vi "AprilTag Target Package Rebound Rumble Code.vi"() -> ()   [LabVIEW 2023]
uses:
  <vilib>/vision/Image Controls.llb/IMAQ Image.ctl
  <vilib>/Utility/config.llb/NI_LVConfig.lvlib
  Camera Set Up/Event/Event Setup Types.ctl
  State Machine/AprialTag States.ctl
  State Machine/AprialTag Main Cluster.ctl
  Steam Type.ctl
  <vilib>/Utility/config.llb/Write Key (String).vi
  <vilib>/Utility/config.llb/Read Key (String).vi
  <vilib>/ptbypt/NI_PtbyPt.lvlib
  <vilib>/vision/NI_Vision_Development_Module.lvlib
  Camera Info.ctl
  <vilib>/vision/Pattern Matching.llb/IMAQ Match Range Setting.ctl
  <vilib>/vision/Shape Detection.llb/ShapeDetectionMatchOptions.ctl
panel:
  in  "Main":enum32{"Page 1", "Page 2"}(tab)
  out "Target Pitch":dbl[](array[numeric]) caption="Tag Pitch (deg)" format="%.1f"
  out "Target Yaw":dbl[](array[numeric]) caption="Tag Yaw (deg)" format="%.1f"
  out "Tag ID":dbl[](array[numeric]) caption="Tag Number"
  out "Image":T1(plugin-control)
  in  "Camera Name":string="cam0"
  in  "Settings":bool
  in  "Save":bool
  in  "Tools":bool
  out "AprilTag Fps":dbl format="%#.0f"
  out "Distance":dbl[](array[numeric]) caption="Tag Distance (in)" format="%.1f"
  out "Angle":dbl[](array[numeric]) caption="Center Angle (deg)" format="%.1f"
  in  "Minimum match score":dbl=100.0
  in  "Home":bool
  in  "Robot Calibration Cluster":T2={"Camera Height on robot (in)"=9.5, "Camera Angle on the robot (deg)"=2.5, "Camera FOV Top to Bottom View Angle (deg)"=26.5, "Camera FOV Left to Right View Angle (deg)"=68.5, "Target size (in)"=6.5, "Distance to front of bumper (in)"=9.75, "Focal Length (mm)"=10.0, "Yaw Slope"=12.276, "Yaw Offset"=2.0} {"Yaw Offset" format="%#_13g"; "Yaw Slope" format="%#_13g"; "Camera FOV Left to Right View Angle (deg)" format="%#_13g"; "Focal Length (mm)" format="%#_13g"; "Distance to front of bumper (in)" format="%#_13g"; "Target size (in)" format="%#_13g"; "Camera FOV Top to Bottom View Angle (deg)" format="%#_13g"; "Camera Angle on the robot (deg)" format="%#_13g"; "Camera Height on robot (in)" format="%#_13g"}
  in  "Max Rect Size (pix)":dbl=1200.0
  in  "Min Rect Size (pix)":dbl=50.0
  in  "Match Options":T3={"Rotation"=TRUE, "Scale"=TRUE, "Occlusion"=FALSE, "Range Settings"=[{"Match Constraints"=0, "Min"=-25.0, "Max"=25.0}, {"Match Constraints"=1, "Min"=25.0, "Max"=200.0}]} {"Range Settings"."Match Constraints" items=["Rotation Angle (degrees)", "Scale Factor (%)", "Occlusion (%)"]}
  # "Edit the camera name to the camera that you are going to use for this target package"
  # "Range"
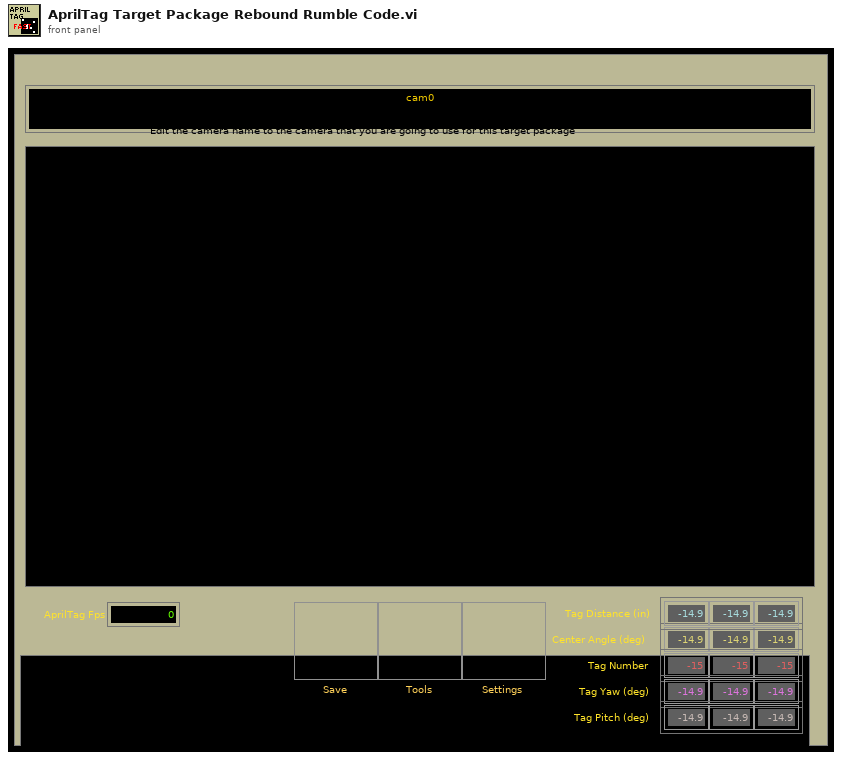
[diagram p1: front panel]
types:
  T1 = typedef "IMAQ Image.ctl" = refnum<image>
  T2 = typedef "Camera Info.ctl" = cluster{"Camera Height on robot (in)":dbl, "Camera Angle on the robot (deg)":dbl, "Camera FOV Top to Bottom View Angle (deg)":dbl, "Camera FOV Left to Right View Angle (deg)":dbl, "Target size (in)":dbl, "Distance to front of bumper (in)":dbl, "Focal Length (mm)":dbl, "Yaw Slope":dbl, "Yaw Offset":dbl}
  T3 = typedef "ShapeDetectionMatchOptions.ctl" = cluster{"Rotation":bool, "Scale":bool, "Occlusion":bool, "Range Settings":T4[]}
  T4 = typedef "IMAQ Match Range Setting.ctl" = cluster{"Match Constraints":u32, "Min":dbl, "Max":dbl}
  T5 = typedef "AprialTag States.ctl" = enum16{"Message Dispatcher", "INI", "Open", "Save", "Exit"}
  T6 = typedef "AprialTag Main Cluster.ctl" = cluster{"AprilTage FIFO":T5[], "Camera Name":string, "AprilTag path":path, "Control Ref's":refnum<vi>[], "Main Image":T1, "Intensity Mask":T1, "Resize Mask":T1, "Timeout":i32, "EDIT Settings":bool, "Calibration path":path, "Camera Number":dbl}
  T7 = cluster{"Min Width":dbl, "Max Width":dbl, "Min Height":dbl, "Max Height":dbl}
  T8 = typedef "Steam Type.ctl" = enum8{"Unknown", "Apriltag", "Algae", "Coral"}
  T9 = typedef "Event Setup Types.ctl" = enum16{"Default", "Camera Loop Started", "Close Settings", "GreyScale", "Open Front Panel", "Reset Team Number", "Save Data", "Exit"}
  T10 = typedef "AprilTag Target Fields.ctl" = cluster{"diameter points":cluster{"first point":cluster{"x":dbl, "y":dbl}, "projected point":cluster{"x":dbl, "y":dbl}}, "normalized center":cluster{"x":dbl, "y":dbl}, "Overall Score":dbl, "Distance (ft)":dbl, "Offset Angle":dbl, "Tag corner points":cluster{"X":dbl, "Y":dbl}[], "Tag Center":cluster{"X":dbl, "Y":dbl}, "Tag Yaw":dbl, "Tag Pitch":dbl, "Target Roll (deg)":dbl, "AprilTag Number":i32, "homography matrix":dbl[]}
  T11 = typedef "Image Type" = u32
  T12 = typedef "NI_LVConfig.lvlib/Config Data RefNum.ctl" = refnum<k1>
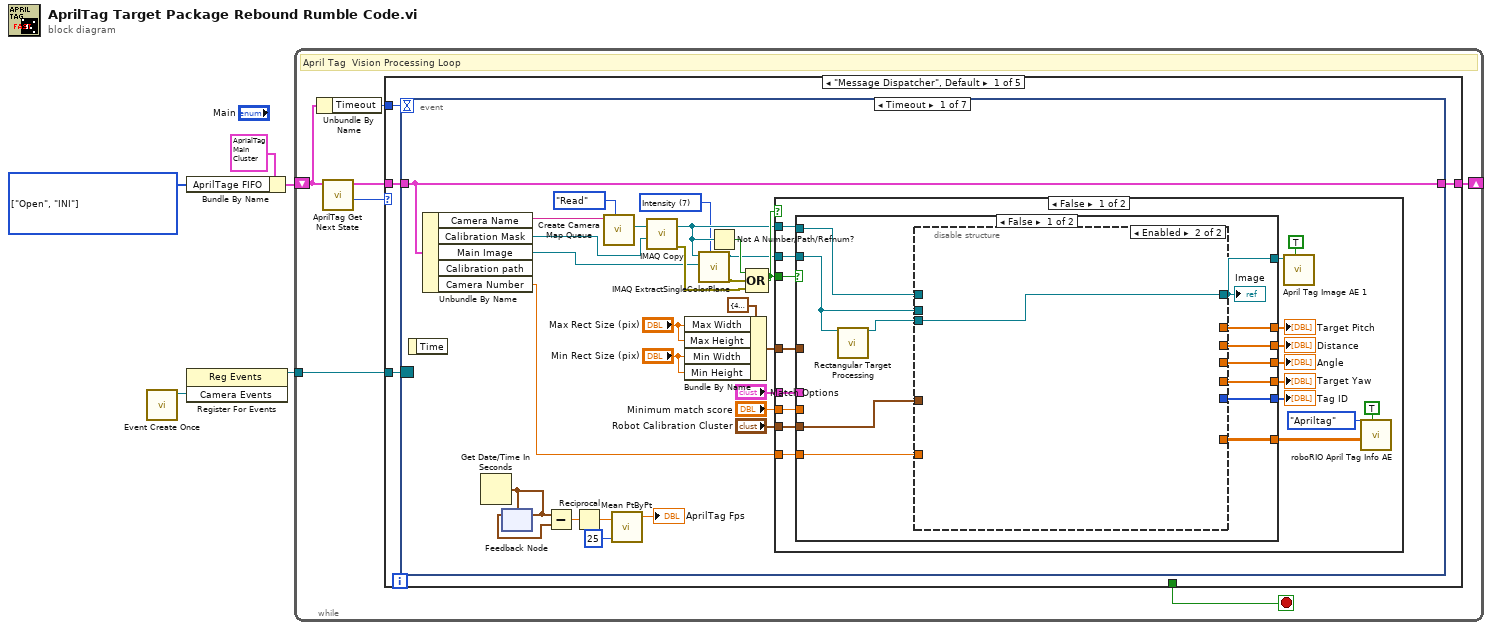
[diagram p0: block diagram]
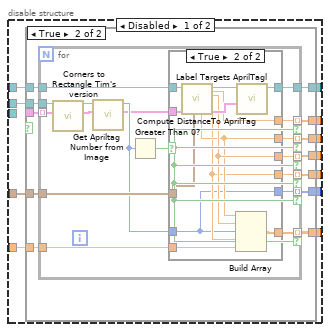
[diagram p2: hidden frame]
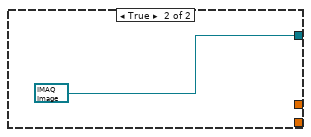
[diagram p5: hidden frame]
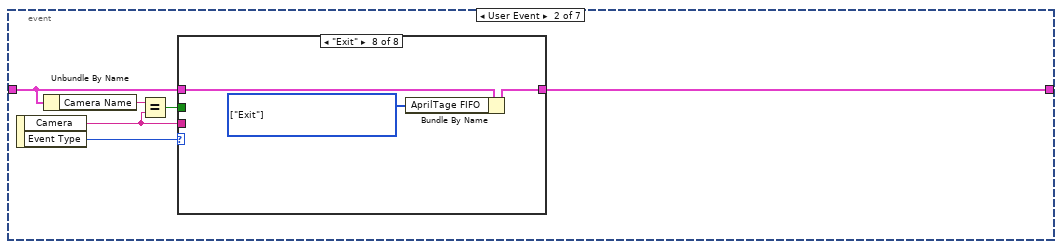
[diagram p7: hidden frame]
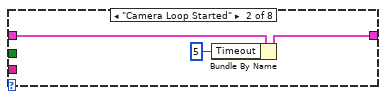
[diagram p9: hidden frame]
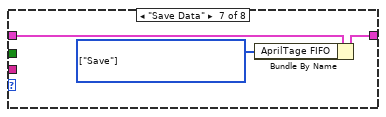
[diagram p14: hidden frame]
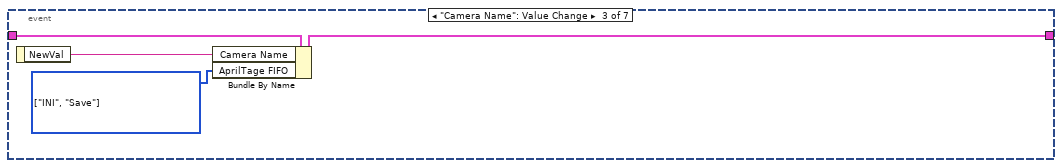
[diagram p15: hidden frame]
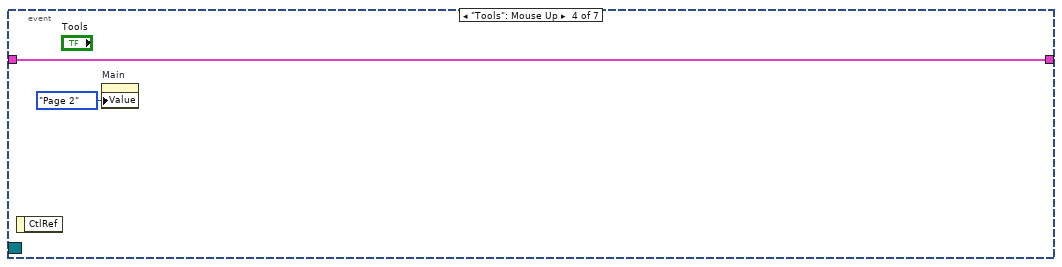
[diagram p16: hidden frame]
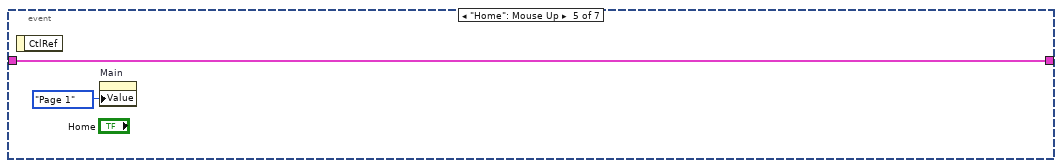
[diagram p17: hidden frame]
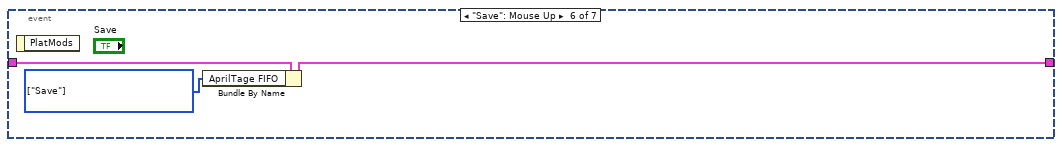
[diagram p18: hidden frame]
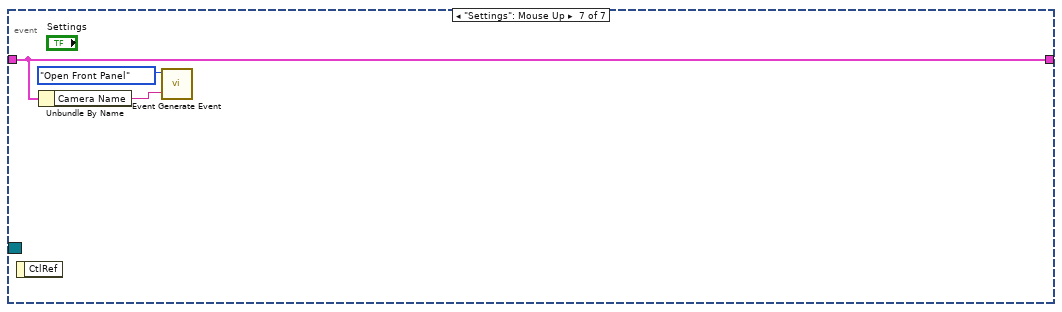
[diagram p19: hidden frame]
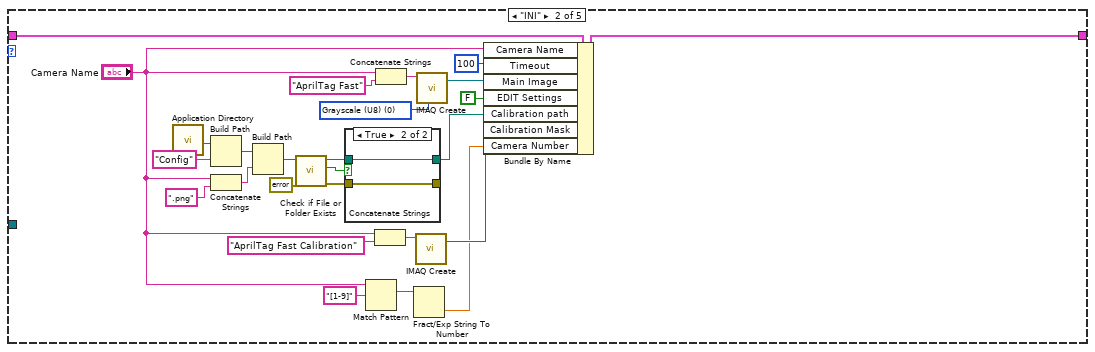
[diagram p20: hidden frame]
diagram:
  w1 = T5[] [enum."Open", enum."INI"] items=["Message Dispatcher", "INI", "Open", "Save", "Exit"] ("AprilTage FIFO")
  n1 = call "Event Create Once.vi"() -> ("Camera Events"=w5:refnum<user-event>)  [unwired: 10 in, 1 out]
  n2 = Bundle By Name(cluster=T6 {"AprilTage FIFO"=[], "Camera Name"="", "AprilTag path"=path "", "Control Ref's"=[], "Main Image"=refnum, "Intensity Mask"=refnum, "Resize Mask"=refnum, "Timeout"=5, "EDIT Settings"=FALSE, "Calibration path"=path "", "Camera Number"=0.0} ("AprilTag Main Cluster out"), "AprilTage FIFO"=w1) -> (w2:T6)
  n3 = register-events(w5) -> (reference out=w4:refnum<event-registration>)  [unwired: 2 in, 1 out]
  n4 = while {
    tunnel: w4 -> [w12]
    shift-right: [w8] -> _
    shift-left: w2 -> [w6]
    stop <- w11 stop-if-true
    # "April Tag  Vision Processing Loop"
    n5 = Unbundle By Name(w6) -> ("Timeout"=w7:i32)
    n6 = call "AprilTag Get Next State.vi"("AprilTag Main Cluster in"=w6) -> ("Next State"=w9:T5, "AprilTag Main Cluster out"=w10:T6)  [unwired: 9 in]
    n7 = case shown="\"Message Dispatcher\", Default" w9 {
      tunnel: w12 -> [w16 _ _ _ _]
      tunnel: [_ _ _ _ TRUE] -> w11
      tunnel: w10 -> [w14 w189 w210 w248 w265]
      tunnel: [w15 w188 w208 w248 w265] -> w8
      tunnel: w7 -> [w13 _ _ _ _]
      frame "Message Dispatcher", Default {
        n8 = event shown="[0] Timeout" {
          selector: w16 -> [_ _ _ _ _ _ _]
          dyn-events: _ -> [_ _ _ _ _ _ _]
          timeout: w13 -> [_ _ _ _ _ _ _]
          tunnel: w14 -> [w43 w133 w153 w154 w156 w160 w162]
          tunnel: [w43 w135 w152 w154 w156 w159 w162] -> w15
          event Timeout {
            w18 = 7 items=["Red", "Green", "Blue", "Hue", "Saturation", "Luminance", "Value", "Intensity"] ("Color Plane")
            n9 = event-data() -> ()  [unwired: 1 in, 1 out]
            n10 = Unbundle By Name(w43) -> ("Camera Name"=w41:string, "Calibration Mask"=w23:T1, "Main Image"=w20:T1, "Camera Number"=w40:dbl)  [unwired: 1 out]
            n11 = Get Date/Time In Seconds() -> (seconds since 1Jan1904=w29:timestamp)
            n12 = feedback-in #1(w29) -> ()
            n13 = feedback #1(w29) -> (w30:timestamp)
            n14 = Subtract(x=w29, y=w30) -> (x-y=w28:dbl)
            n15 = Reciprocal(x=w28) -> (1/x=w27:dbl)
            n16 = call "Create Camera Map Queue.vi"("Action"=enum16{"Read", "Write"}."Read", "Camera"=w41) -> ("Image out"=w24:T1)  [unwired: 8 in, 1 out]
            n17 = call <vilib>:"Mean PtByPt.vi"("x"=w27, "sample length"=25) -> ("mean"=→"AprilTag Fps":dbl)  [unwired: 2 in, 1 out]
            n18 = call "IMAQ Copy"("Image Dst"=w23, "Image Src"=w24) -> ("error out"=w22:errorcluster, "Image Dst Out"=w21:T1)  [unwired: 4 in]
            n19 = Bundle By Name(cluster=T7 {"Min Width"=40.0, "Max Width"=100.0, "Min Height"=40.0, "Max Height"=200.0} ("Rectangle Descriptor"), "Max Width"="Max Rect Size (pix)", "Max Height"="Max Rect Size (pix)", "Min Width"="Min Rect Size (pix)", "Min Height"="Min Rect Size (pix)") -> (w39:T7)
            n20 = call "IMAQ ExtractSingleColorPlane"("Color Plane"=w18, "Image Dst"=w20, "Image Src"=w21) -> ("error out"=w17:errorcluster, "Image Dst Out"=w19:T1)  [unwired: 7 in]
            n21 = Not A Number/Path/Refnum?(number/path/refnum=w21) -> (NaN/Path/Refnum?=w32:bool)
            n22 = Compound Arithmetic op=OR(w32, w17, w22) -> (w31:bool)
            n23 = case shown="False" w31 {
              tunnel: "Robot Calibration Cluster" -> [w58 _]
              tunnel: w31 -> [w52 _]
              tunnel: w21 -> [w51 _]
              tunnel: w40 -> [w50 _]
              tunnel: w39 -> [w48 _]
              tunnel: "Match Options" -> [w47 _]
              tunnel: w19 -> [w46 _]
              tunnel: "Minimum match score" -> [w45 _]
              frame False {
                n24 = case shown="False" w52 {
                  tunnel: w58 -> [w73 _]
                  tunnel: [w72 _] -> w60
                  tunnel: [w71 _] -> w57
                  tunnel: [w70 _] -> w56
                  tunnel: [w69 _] -> w55
                  tunnel: [w68 _] -> w54
                  tunnel: [w67 _] -> w53
                  tunnel: w51 -> [w64 _]
                  tunnel: w50 -> [w66 _]
                  tunnel: [w65 T1 refnum ("Image out")] -> w49
                  tunnel: w48 -> [_ _]
                  tunnel: w47 -> [_ _]
                  tunnel: w46 -> [w62 _]
                  tunnel: w45 -> [_ _]
                  frame False {
                    n25 = call "Rectangular Target Processing.vi"("Original Image"=w62) -> ("Processed Image"=w63:T1)  [unwired: 13 in, 1 out]
                    n26 = disable-structure shown="Enabled" {
                      disable-tunnel: w73 -> [w84 _]
                      disable-tunnel: [w83 _] -> w72
                      disable-tunnel: [w82 _] -> w71
                      disable-tunnel: [w81 _] -> w70
                      disable-tunnel: [w80 _] -> w69
                      disable-tunnel: [w79 _] -> w68
                      disable-tunnel: [w78 _] -> w67
                      disable-tunnel: w66 -> [w77 _]
                      disable-tunnel: [w76 w128] -> w65
                      disable-tunnel: w62 -> [w75 _]
                      disable-tunnel: w64 -> [w74 _]
                      disable-tunnel: w63 -> [_ w128]
                      frame Disabled {
                        n27 = case shown="True" {
                          selector: _ -> [_ _]
                          tunnel: w74 -> [w85 w86]
                          tunnel: _ -> [_ w97]
                          tunnel: [w85 w88] -> w76
                          tunnel: w84 -> [_ w96]
                          tunnel: [_ w95] -> w83
                          tunnel: [_ w94] -> w82
                          tunnel: [_ w93] -> w81
                          tunnel: [_ w92] -> w80
                          tunnel: [_ w91] -> w79
                          tunnel: [_ w90] -> w78
                          tunnel: w77 -> [_ w89]
                          tunnel: w75 -> [_ w87]
                          frame False {
                          }
                          frame True {
                            n28 = for {
                              tunnel: w97 -> [w112] mode=indexing
                              tunnel: w86 -> [w104]
                              tunnel: [w113] -> w88
                              tunnel: [w98] -> w92 mode=indexing if=w99
                              tunnel: [w109] -> w90 mode=indexing if=w99
                              tunnel: [w111] -> w91 mode=indexing if=w99
                              tunnel: w96 -> [w110]
                              tunnel: [w108] -> w93 mode=indexing if=w99
                              tunnel: [w107] -> w95 mode=indexing if=w99
                              tunnel: [w106] -> w94 mode=indexing if=w99
                              tunnel: w89 -> [w105]
                              tunnel: w87 -> [w102]
                              n29 = call "Corners to Rectangle Tim's version.vi"("Rectangle Descriptor"=w112) -> ("tag info out"=w101:T10)  [unwired: 10 in]
                              n30 = call "Get Apriltag Number from Image.vi"("tag info"=w101, "Image"=w102) -> ("tag info out"=w100:T10, "AprilTag#"=w103:i32)  [unwired: 7 in, 1 out]
                              n31 = Greater Than 0?(x=w103) -> (x > 0?=w99:bool)
                              n32 = case shown="True" w99 {
                                tunnel: [w114 w127] -> w113
                                tunnel: w100 -> [_ w126]
                                tunnel: [_ w123] -> w111
                                tunnel: w110 -> [_ w122]
                                tunnel: [_ w121] -> w109
                                tunnel: [_ w120] -> w108
                                tunnel: [_ w119] -> w107
                                tunnel: [_ w118] -> w106
                                tunnel: w105 -> [_ w117]
                                tunnel: w104 -> [w114 w116]
                                tunnel: w103 -> [_ w115]
                                tunnel: [_ w115] -> w98
                                frame False {
                                }
                                frame True {
                                n33 = call "Compute DistanceTo AprilTag.vi"("Robot Calibration Cluster"=w122, "results"=w126, "Image Src"=w116) -> ("results out"=w125:T10, "Target Yaw (deg)"=w120:dbl, "Offset Angle"=w123:dbl, "Image Dst Out"=w124:T1, "Distance from target (in)"=w121:dbl, "Target Pitch (deg)"=w118:dbl)  [unwired: 2 in, 1 out]
                                n34 = Build Array(w121, w123, w115, w120, w117) -> (w119:dbl[])
                                n35 = call "Label Targets AprilTagl.vi"("results"=w125, "Image in"=w124) -> ("Image out"=w127:T1)  [unwired: 9 in]
                                }
                              }
                            }
                          }
                        }
                      }
                      frame Enabled {
                      }
                    }
                    "Image" <- w65
                  }
                  frame True {
                  }
                }
                "Distance" <- w53
                "Angle" <- w54
                "Tag ID" <- w55
                "Target Yaw" <- w56
                "Target Pitch" <- w57
                n36 = call "April Tag Image AE 1.vi"("Update"=TRUE, "Ball Image in"=w49) -> ()  [unwired: 9 in, 1 out]
                n37 = call "roboRIO April Tag Info AE.vi"("Update"=TRUE, "Info in"=w60, "Stream Type"=Steam_Type."Apriltag") -> ()  [unwired: 8 in, 1 out]
              }
              frame True {
              }
            }
          }
          event User Event {
            n38 = event-data() -> ("Camera"=w130:string, "Event Type"=w134:T9)  [unwired: 1 in]
            n39 = Unbundle By Name(w133) -> ("Camera Name"=w132:string)
            n40 = Equal?(x=w132, y=w130) -> (x = y?=w131:bool)
            n41 = case shown="\"Exit\"" w134 {
              tunnel: w133 -> [w136 w139 w140 w141 w142 w143 w146 w149]
              tunnel: [w136 w138 w140 w141 w142 w143 w145 w148] -> w135
              tunnel: w131 -> [_ _ _ _ _ _ _ _]
              tunnel: w130 -> [_ _ _ _ _ _ _ _]
              frame "Default" {
              }
              frame "Camera Loop Started" {
                n42 = Bundle By Name(cluster=w139, "Timeout"=5) -> (w138:T6)
              }
              frame "Close Settings" {
              }
              frame "GreyScale" {
              }
              frame "Open Front Panel" {
              }
              frame "Reset Team Number" {
              }
              frame "Save Data" {
                w144 = T5[] [enum."Save"] items=["Message Dispatcher", "INI", "Open", "Save", "Exit"] ("AprilTage FIFO")
                n43 = Bundle By Name(cluster=w146, "AprilTage FIFO"=w144) -> (w145:T6)
              }
              frame "Exit" {
                w147 = T5[] [enum."Exit"] items=["Message Dispatcher", "INI", "Open", "Save", "Exit"] ("AprilTage FIFO")
                n44 = Bundle By Name(cluster=w149, "AprilTage FIFO"=w147) -> (w148:T6)
              }
            }
          }
          event "Camera Name": Value Change {
            w151 = T5[] [enum."INI", enum."Save"] items=["Message Dispatcher", "INI", "Open", "Save", "Exit"] ("AprilTage FIFO")
            n45 = event-data() -> ("NewVal"=w150:string)  [unwired: 1 in]
            n46 = Bundle By Name(cluster=w153, "Camera Name"=w150, "AprilTage FIFO"=w151) -> (w152:T6)
          }
          event "Tools": Mouse Up {
            n47 = event-data() -> ()  [unwired: 1 in, 1 out]
            n48 = property on="Main" class="TabCtl (strict)"("Value"=enum32{"Page 1", "Page 2"}."Page 2" ("Main")) -> ()  [unwired: 2 in, 2 out]
          }
          event "Home": Mouse Up {
            n49 = event-data() -> ()  [unwired: 1 in, 1 out]
            n50 = property on="Main" class="TabCtl (strict)"("Value"=enum32{"Page 1", "Page 2"}."Page 1" ("Main")) -> ()  [unwired: 2 in, 2 out]
          }
          event "Save": Mouse Up {
            w158 = T5[] [enum."Save"] items=["Message Dispatcher", "INI", "Open", "Save", "Exit"] ("AprilTage FIFO")
            n51 = event-data() -> ()  [unwired: 1 in, 1 out]
            n52 = Bundle By Name(cluster=w160, "AprilTage FIFO"=w158) -> (w159:T6)
          }
          event "Settings": Mouse Up {
            n53 = event-data() -> ()  [unwired: 1 in, 1 out]
            n54 = Unbundle By Name(w162) -> ("Camera Name"=w161:string)
            n55 = call "Event Generate Event.vi"("Camera Name"=w161, "Event Type"=Event_Setup_Types."Open Front Panel") -> ()  [unwired: 10 in]
          }
        }
      }
      frame "INI" {
        w186 = T11 0 items=["Grayscale (U8)", "Grayscale (I16)", "Grayscale (SGL)", "Complex (CSG)", "RGB (U32)", "HSL (U32)", "RGB (U64)", "Grayscale (U16)"] ("Image Type")
        n56 = call <vilib>:"Application Directory.vi"() -> ("Application Directory"=w179:path)
        n57 = Build Path(base path=w179, name or relative path="Config") -> (appended path=w177:path)
        n58 = Concatenate Strings("Camera Name", ".png" ("name or relative path")) -> (w181:string)
        n59 = Build Path(base path=w177, name or relative path=w181) -> (appended path=w176:path)
        n60 = call <vilib>:"Check if File or Folder Exists.vi"("error in (no error)"=errorcluster {"status"=FALSE, "code"=0, "source"=""}, "path"=w176) -> ("error out"=w173:errorcluster, "file or folder exists?"=w174:bool, "dup path"=w175:path)  [unwired: 7 in]
        n61 = case shown="True" w174 {
          tunnel: [w192 w193] -> _
          tunnel: w175 -> [w191 w194]
          tunnel: [w191 w194] -> w171
          tunnel: w173 -> [w190 w193]
          frame False {
            n62 = call <vilib>:"Create File and Containing Folders.vi"("error in (no error)"=w190, "file path"=w191) -> ("error out"=w192:errorcluster)  [unwired: 8 in, 1 out]
          }
          frame True {
          }
        }
        n63 = Match Pattern(string="Camera Name", regular expression="[1-9]") -> (match substring=w166:string)  [unwired: 1 in, 3 out]
        n64 = Concatenate Strings("Camera Name", "AprilTag Fast Calibration" ("string")) -> (w169:string)
        n65 = Concatenate Strings("Camera Name", "AprilTag Fast" ("string")) -> (w185:string)
        n66 = Fract/Exp String To Number(string=w166) -> (number=w165:dbl)  [unwired: 3 in, 1 out]
        n67 = call "IMAQ Create"("Image Name"=w169) -> ("New Image"=w168:T1)  [unwired: 3 in, 2 out]
        n68 = call "IMAQ Create"("Image Name"=w185, "Image Type"=w186) -> ("New Image"=w183:T1)  [unwired: 2 in, 2 out]
        n69 = Bundle By Name(cluster=w189, "Camera Name"="Camera Name", "Timeout"=100, "Main Image"=w183, "EDIT Settings"=FALSE, "Calibration path"=w171, "Calibration Mask"=w168, "Camera Number"=w165) -> (w188:T6)
      }
      frame "Open" {
        n70 = call <vilib>:"Application Directory.vi"() -> ("Application Directory"=w213:path)
        n71 = Build Path(base path=w213, name or relative path="Config") -> (appended path=w211:path)
        n72 = Concatenate Strings("Airtag1" ("string"), ".ini" ("name or relative path")) -> (w223:string)
        n73 = Build Path(base path=w211, name or relative path=w223) -> (appended path=w204:path)
        n74 = call <vilib>:"Check if File or Folder Exists.vi"("error in (no error)"=errorcluster {"status"=FALSE, "code"=0, "source"=""}, "path"=w204) -> ("error out"=w200:errorcluster, "file or folder exists?"=w202:bool, "dup path"=w203:path)  [unwired: 7 in]
        n75 = control-ref of="Main"() -> (w218:refnum<vi>)
        n76 = case shown="False" w202 {
          tunnel: [w226 w227] -> w214
          tunnel: w203 -> [w225 w228]
          tunnel: [w225 w228] -> w201
          tunnel: w200 -> [w224 w227]
          frame False {
            n77 = call <vilib>:"Create File and Containing Folders.vi"("error in (no error)"=w224, "file path"=w225) -> ("error out"=w226:errorcluster)  [unwired: 8 in, 1 out]
          }
          frame True {
          }
        }
        n78 = control-ref of="Robot Calibration Cluster"() -> (w217:refnum<vi>)
        n79 = control-ref of="Match Options"() -> (w198:refnum<vi>)
        n80 = control-ref of="Minimum match score"() -> (w197:refnum<vi>)
        n81 = control-ref of="Max Rect Size (pix)"() -> (w196:refnum<vi>)
        n82 = control-ref of="Min Rect Size (pix)"() -> (w195:refnum<vi>)
        n83 = control-ref of="Camera Name"() -> (w209:refnum<vi>)
        n84 = Build Array(w218, w217, w209, w198, w197, w196, w195) -> (w207:refnum<vi>[])
        n85 = call <vilib>:"Open Config Data.vi"("error in (no error)"=w214, "configuration file path"=w201) -> ("error out"=w219:errorcluster, "refnum"=w222:T12)  [unwired: 7 in, 1 out]
        n86 = for {
          tunnel: "Info" ("Camera Name") -> [w241]
          tunnel: w207 -> [w239] mode=indexing
          shift-right: [w243] -> w221
          shift-left: w222 -> [w244]
          shift-right: [w242] -> w220
          shift-left: w219 -> [w240]
          tunnel: [w234] -> _ mode=indexing
          tunnel: errorcluster {"status"=FALSE, "code"=0, "source"=""} ("error out") -> [w233]
          tunnel: [w229] -> _ mode=indexing
          n87 = property class="Ctl"(reference=w239, error in=w233) -> (reference out=w237:refnum<vi>, error out=w235:errorcluster, "Label.Text"=w238:string, "Value"=w231:variant)
          n88 = Variant To Flattened String(Variant=w231) -> (1:w230:i16[])  [unwired: 1 out]
          n89 = call-poly <vilib>:"Read Key.vi"("section"=w241, "error in (no error)"=w240, "key"=w238, "refnum"=w244) -> ("error out"=w242:errorcluster, "value"=w236:string, "refnum out"=w243:T12)  [unwired: 4 in, 1 out]
          n90 = Flattened String To Variant(6:w236, 7:w230) -> (0:w229:errorcluster, 3:w232:variant)  [unwired: 1 in]
          n91 = property class="Ctl"(reference=w237, error in=w235, "Value"=w232) -> (error out=w234:errorcluster)  [unwired: 1 out]
        }
        n92 = call <vilib>:"Close Config Data.vi"("error in (no error)"=w220, "refnum"=w221) -> ()  [unwired: 8 in, 2 out]
        n93 = Bundle By Name(cluster=w210, "Control Ref's"=w207, "AprilTag path"=w201) -> (w208:T6)
      }
      frame "Save" {
        n94 = Unbundle By Name(w248) -> ("Control Ref's"=w246:refnum<vi>[], "AprilTag path"=w247:path)
        n95 = call <vilib>:"Open Config Data.vi"("configuration file path"=w247) -> ("error out"=w249:errorcluster, "refnum"=w252:T12)  [unwired: 8 in, 1 out]
        n96 = for {
          tunnel: "Info" ("Camera Name") -> [w258]
          shift-right: [w261] -> w251
          shift-left: w252 -> [w262]
          shift-right: [w260] -> w250
          shift-left: w249 -> [w259]
          tunnel: w246 -> [w253] mode=indexing
          n97 = property class="Ctl"(reference=w253, error in=w259) -> (error out=w255:errorcluster, "Label.Text"=w257:string, "Value"=w256:variant)  [unwired: 1 out]
          n98 = Variant To Flattened String(Variant=w256) -> (data string=w254:string)  [unwired: 1 out]
          n99 = call-poly <vilib>:"Write Key.vi"("section"=w258, "error in (no error)"=w255, "value"=w254, "key"=w257, "refnum"=w262) -> ("error out"=w260:errorcluster, "refnum out"=w261:T12)  [unwired: 4 in, 1 out]
        }
        n100 = call <vilib>:"Close Config Data.vi"("error in (no error)"=w250, "refnum"=w251) -> ()  [unwired: 8 in, 2 out]
      }
      frame "Exit" {
        n101 = Unbundle By Name(w265) -> ("Calibration Mask"=w264:T1, "Main Image"=w263:T1)
        n102 = call "IMAQ Dispose"("Image"=w264) -> ()  [unwired: 5 in, 1 out]
        n103 = call "IMAQ Dispose"("Image"=w263) -> ()  [unwired: 5 in, 1 out]
      }
    }
  }
